vi "HallSafety.vi"   [LabVIEW 2015]
uses:
  Robot Global Data.vi
types:
  T1 = typedef "WPI_MotorControlDeviceRef.ctl" = cluster{"DeviceStatus":errorcluster, "Type":T2, "PWM":cluster{"PWM Channel":T3, "DeadBand":T4}, "CAN":cluster{"Device Number":u8, "Control Mode":T5, "Semaphore":T6, "Max Vout":dbl, "TalonSRX Control Mode":T7}, "Invert":bool}
  T2 = typedef "WPI_MotorControlType.ctl" = enum16{"PWM", "CAN", "CANTalonSRX"}
  T3 = typedef "FPGA_DIOPWMChannel.ctl" = enum8{"PWM 0", "PWM 1", "PWM 2", "PWM 3", "PWM 4", "PWM 5", "PWM 6", "PWM 7", "PWM 8", "PWM 9", "PWM MXP 0", "PWM MXP 1", "PWM MXP 2", "PWM MXP 3", "PWM MXP 4", "PWM MXP 5", "PWM MXP 6", "PWM MXP 7", "PWM MXP 8", "PWM MXP 9", "Invalid"}
  T4 = typedef "WPI_PWMDeadband.ctl" = cluster{"Name":string, "maxPositivePwm":i32, "minPositivePwm":i32, "centerPwm":i32, "maxNegativePwm":i32, "minNegativePwm":i32, "angularRange":u16}
  T5 = typedef "WPI_CANJaguar_ControlMode.ctl" = enum8{"Percent VBus", "Current", "Speed", "Position", "Voltage"}
  T6 = typedef "Semaphore RefNum" = refnum<k1>
  T7 = typedef "WPI_CANTalonSRX_APIControlMode.ctl" = enum8{"Percent VBus", "Speed", "Position", "Slave", "Unchanged / Invalid", "Voltage Compensation", "Current", "Motion Profile"}
  T8 = typedef "WPI_DigitalInputDevRef.ctl" = cluster{"DevStatus":errorcluster, "DIO Channel":T9}
  T9 = typedef "FPGA_DIOChannel.ctl" = enum8{"DIO 0", "DIO 1", "DIO 2", "DIO 3", "DIO 4", "DIO 5", "DIO 6", "DIO 7", "DIO 8", "DIO 9", "DIO MXP 0", "DIO MXP 1", "DIO MXP 2", "DIO MXP 3", "DIO MXP 4", "DIO MXP 5", "DIO MXP 6", "DIO MXP 7", "DIO MXP 8", "DIO MXP 9", "DIO MXP 10", "DIO MXP 11", "DIO MXP 12", "DIO MXP 13", "DIO MXP 14", "DIO MXP 15", "Invalid"}
  T10 = cluster{"Firing Angle":dbl, "Max Angle?":bool, "Min Angle?":bool}
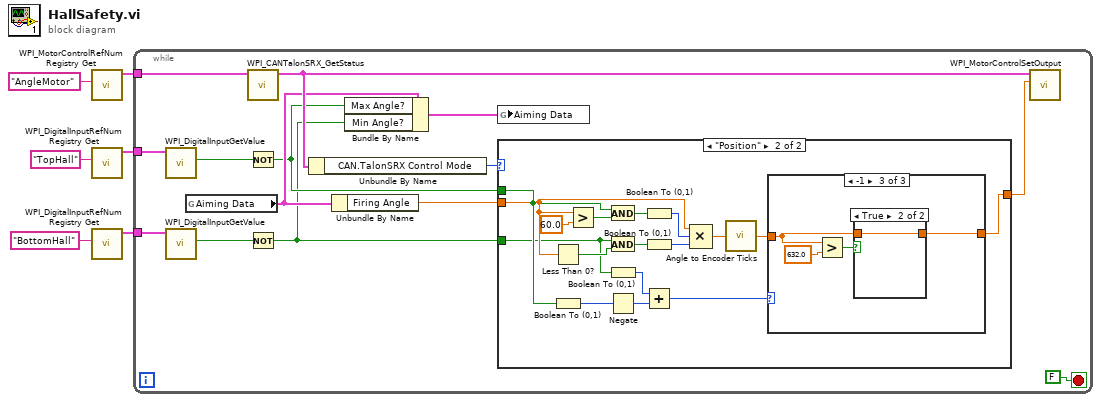
[diagram p0: block diagram]
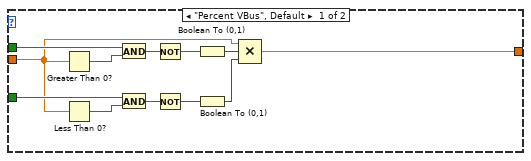
[diagram p2: hidden frame]
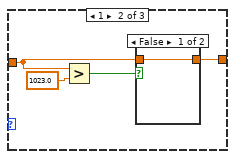
[diagram p4: hidden frame]
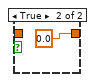
[diagram p5: hidden frame]
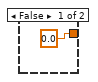
[diagram p6: hidden frame]
diagram:
  n1 = call <vilib>:"WPI_MotorControlRefNum Registry Get.vi"("refnum name"="AngleMotor") -> ("MotorControlDevRef"=w1:T1)  [unwired: 9 in, 1 out]
  n2 = call <vilib>:"WPI_DigitalInputRefNum Registry Get.vi"("refnum name"="TopHall") -> ("DigitalInputDevRef"=w5:T8)  [unwired: 9 in, 1 out]
  n3 = call <vilib>:"WPI_DigitalInputRefNum Registry Get.vi"("refnum name"="BottomHall") -> ("DigitalInputDevRef"=w2:T8)  [unwired: 9 in, 1 out]
  n4 = while {
    tunnel: w5 -> [w17]
    tunnel: w2 -> [w16]
    tunnel: w1 -> [w15]
    stop <- FALSE stop-if-true
    n5 = call <vilib>:"WPI_DigitalInputGetValue.vi"("DigitalInputDevRef"=w17) -> ("Value"=w13:bool)  [unwired: 8 in, 2 out]
    n6 = call <vilib>:"WPI_DigitalInputGetValue.vi"("DigitalInputDevRef"=w16) -> ("Value"=w12:bool)  [unwired: 8 in, 2 out]
    n7 = global read "Robot Global Data.vi" "Aiming Data"() -> (w10:T10)
    n8 = call <vilib>:"WPI_CANTalonSRX_GetStatus.vi"("CAN Talon SRX Ref"=w15) -> ("CAN Talon SRX Ref"=w18:T1)  [unwired: 8 in, 2 out]
    n9 = Not(x=w13) -> (.not. x?=w8:bool)
    n10 = Not(x=w12) -> (.not. x?=w7:bool)
    n11 = Unbundle By Name(w18) -> ("CAN.TalonSRX Control Mode"=w19:T7)
    n12 = Unbundle By Name(w10) -> ("Firing Angle"=w20:dbl)
    n13 = Bundle By Name(cluster=w10, "Max Angle?"=w8, "Min Angle?"=w7) -> (w9:T10)
    n14 = global write "Robot Global Data.vi" "Aiming Data"(w9) -> ()
    n15 = case shown="\"Position\"" w19 {
      tunnel: [w28 w35] -> w11
      tunnel: w8 -> [w27 w34]
      tunnel: w7 -> [w26 w33]
      tunnel: w20 -> [w25 w41]
      frame "Percent VBus", Default {
        n16 = Greater Than 0?(x=w25) -> (x > 0?=w32:bool)
        n17 = Less Than 0?(x=w25) -> (x < 0?=w31:bool)
        n18 = And(x=w27, y=w32) -> (x .and. y?=w24:bool)
        n19 = And(x=w26, y=w31) -> (x .and. y?=w22:bool)
        n20 = Not(x=w24) -> (.not. x?=w23:bool)
        n21 = Not(x=w22) -> (.not. x?=w21:bool)
        n22 = Boolean To (0,1)(Boolean=w23) -> (0, 1=w29:i16)
        n23 = Boolean To (0,1)(Boolean=w21) -> (0, 1=w30:i16)
        n24 = Compound Arithmetic op=MULTIPLY(w25, w29, w30) -> (w28:dbl)
      }
      frame "Position" {
        n25 = Less Than 0?(x=w41) -> (x < 0?=w48:bool)
        n26 = Boolean To (0,1)(Boolean=w34) -> (0, 1=w37:i16)
        n27 = Greater?(x=w41, y=60.0) -> (0:w49:bool)
        n28 = And(x=w34, y=w49) -> (x .and. y?=w47:bool)
        n29 = And(x=w33, y=w48) -> (x .and. y?=w46:bool)
        n30 = Boolean To (0,1)(Boolean=w33) -> (0, 1=w39:i16)
        n31 = Negate(x=w37) -> (-x=w38:i16)
        n32 = Boolean To (0,1)(Boolean=w47) -> (0, 1=w44:i16)
        n33 = Boolean To (0,1)(Boolean=w46) -> (0, 1=w45:i16)
        n34 = Add(x=w39, y=w38) -> (x+y=w40:i16)
        n35 = Compound Arithmetic op=MULTIPLY(w41, w44, w45) -> (w43:dbl)
        n36 = call "Angle to Encoder Ticks.vi"("Angle(degrees)"=w43) -> ("Pot Data"=w36:dbl)
        n37 = case shown="-1" w40 {
          tunnel: w36 -> [w50 w51 w58]
          tunnel: [w50 w52 w57] -> w35
          frame 0, Default {
          }
          frame 1 {
            n38 = Greater?(x=w51, y=1023.0) -> (0:w53:bool)
            n39 = case shown="False" w53 {
              tunnel: [w55 0.0] -> w52
              tunnel: w51 -> [w55 _]
              frame False {
              }
              frame True {
              }
            }
          }
          frame -1 {
            n40 = Greater?(x=w58, y=632.0) -> (0:w60:bool)
            n41 = case shown="True" w60 {
              tunnel: [0.0 w62] -> w57
              tunnel: w58 -> [_ w62]
              frame False {
              }
              frame True {
              }
            }
          }
        }
      }
    }
    n42 = call <vilib>:"WPI_MotorControlSetOutput.vi"("Output"=w11, "MotorControlDevRef"=w18) -> ()  [unwired: 7 in, 3 out]
  }
